vi "Post-Build Action.vi"(5 "Files Generated by Build":path[](array[path]), 6 "Top Level/Always Included VIs":path[](array[path]), 7 "Destination Path":path, 8 "error in (no error)":errorcluster, 9 "Target Name":string, 10 "Build Specification Name":string, 11 "Project Path":path) -> (0 "error out":errorcluster)   [LabVIEW 2019]
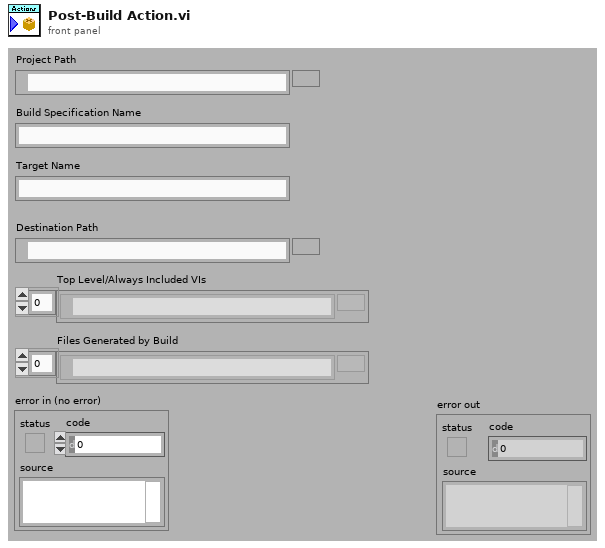
[diagram p1: front panel]
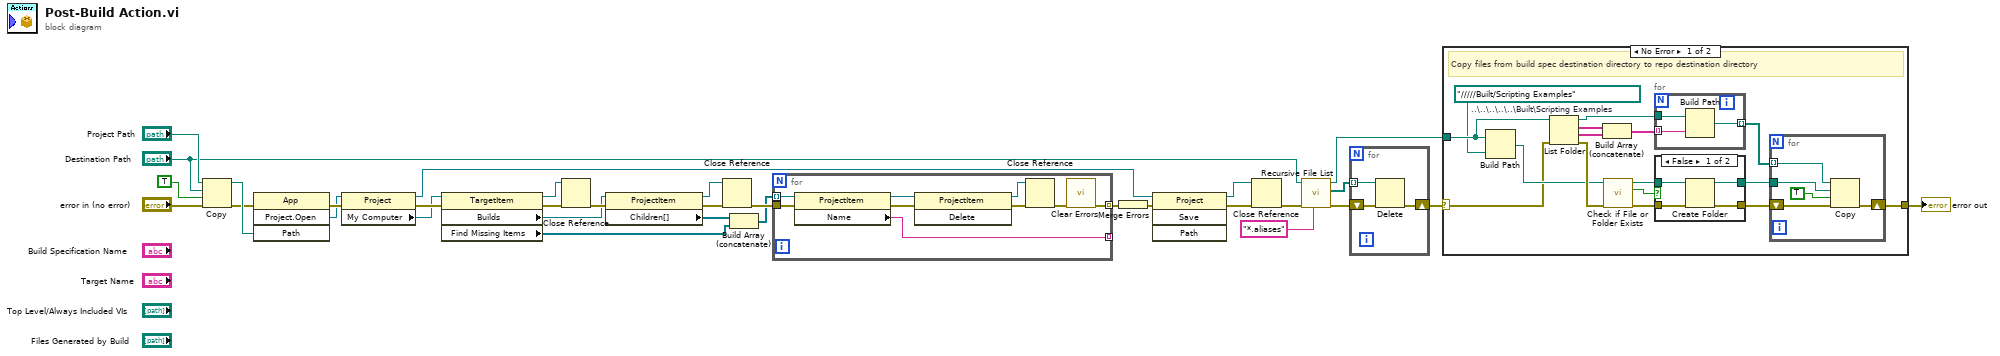
[diagram p0: block diagram]
diagram:
  n1 = Copy(8:"error in (no error)", 9:TRUE ("overwrite (F)"), 10:"Destination Path", 11:"Project Path") -> (0:w22:errorcluster, 3:w26:path)  [unwired: 1 in, 1 out]
  n2 = invoke class="App" method="Project.Open"(error in=w22, "Path"=w26) -> (error out=w23:errorcluster, "Project:Open"=w19:refnum<vi>)  [unwired: 2 in, 2 out]
  n3 = property class="Project"(reference=w19, error in=w23) -> (reference out=w25:refnum<vi>, error out=w24:errorcluster, "My Computer"=w18:refnum<vi>)
  n4 = property class="TargetItem"(reference=w18, error in=w24) -> (reference out=w6:refnum<vi>, error out=w7:errorcluster, "Builds"=w4:refnum<vi>, "Find Missing Items"=w2:refnum<vi>[])
  n5 = Close Reference(reference=w6, error in (no error)=w7) -> (error out=w5:errorcluster)
  n6 = property class="ProjectItem"(reference=w4, error in=w5) -> (reference out=w9:refnum<vi>, error out=w10:errorcluster, "Children[]"=w3:refnum<vi>[])
  n7 = Close Reference(reference=w9, error in (no error)=w10) -> (error out=w8:errorcluster)
  n8 = Build Array (concatenate)(w3, w2) -> (w1:refnum<vi>[])
  n9 = for {
    tunnel: w1 -> [w37] mode=indexing
    tunnel: [w35] -> _ mode=indexing
    tunnel: w8 -> [w39]
    tunnel: [w33] -> w11 mode=indexing
    n10 = property class="ProjectItem"(reference=w37, error in=w39) -> (reference out=w36:refnum<vi>, error out=w38:errorcluster, "Name"=w35:string)
    n11 = invoke class="ProjectItem" method="Delete"(reference=w36, error in=w38) -> (reference out=w40:refnum<vi>, error out=w41:errorcluster)  [unwired: 1 in, 1 out]
    n12 = Close Reference(reference=w40, error in (no error)=w41) -> (error out=w34:errorcluster)
    n13 = call <vilib>:"Clear Errors.vi"("error in (no error)"=w34) -> ("error out"=w33:errorcluster)  [unwired: 5 in, 1 out]
  }
  n14 = Merge Errors(w11) -> (w13:errorcluster)
  n15 = invoke class="Project" method="Save"(reference=w25, error in=w13) -> (reference out=w20:refnum<vi>, error out=w21:errorcluster)  [unwired: 2 in, 2 out]
  n16 = Close Reference(reference=w20, error in (no error)=w21) -> (error out=w17:errorcluster)
  n17 = call <vilib>:"Recursive File List.vi"("pattern"="*.aliases", "error in (no error)"=w17, "Folder Path"="Destination Path") -> ("error out"=w15:errorcluster, "All Files in Dir"=w14:path[], "dup Folder Path"=w28:path)  [unwired: 4 in, 2 out]
  n18 = for {
    shift-right: [w42] -> w27
    shift-left: w15 -> [w44]
    tunnel: w14 -> [w43] mode=indexing
    n19 = Delete(path (use dialog)=w43, error in=w44) -> (error out=w42:errorcluster)  [unwired: 3 in, 2 out]
  }
  n20 = case shown="No Error" w27 {
    selector: w27 -> [w47 w75]
    tunnel: [w58 w75] -> w12
    tunnel: w28 -> [w46 _]
    frame No Error {
      w45 = path "../../../../../Built/Scripting Examples"  # ..\..\..\..\..\Built\Scripting Examples
      # "Copy files from build spec destination directory to repo destination directory"
      n21 = Build Path(base path=w46, name or relative path=w45) -> (appended path=w53:path)
      n22 = List Folder(path=w46, error in=w47) -> (path out=w60:path, filenames=w57:string[], folder names=w56:string[], error out=w59:errorcluster)  [unwired: 2 in]
      n23 = Build Array (concatenate)(w57, w56) -> (w55:string[])
      n24 = call <vilib>:"Check if File or Folder Exists.vi"("error in (no error)"=w59, "path"=w53) -> ("error out"=w50:errorcluster, "file or folder exists?"=w52:bool, "dup path"=w51:path)  [unwired: 7 in]
      n25 = for {
        tunnel: w55 -> [w73] mode=indexing
        tunnel: w60 -> [w74]
        tunnel: [w72] -> w54 mode=indexing
        n26 = Build Path(base path=w74, name or relative path=w73) -> (appended path=w72:path)
      }
      n27 = case shown="False" w52 {
        tunnel: w51 -> [w64 w66]
        tunnel: w50 -> [w63 w65]
        tunnel: [w62 w66] -> w49
        tunnel: [w61 w65] -> w48
        frame False {
          n28 = Create Folder(path (use dialog)=w64, error in=w63) -> (created path=w62:path, error out=w61:errorcluster)  [unwired: 1 in, 1 out]
        }
        frame True {
        }
      }
      n29 = for {
        tunnel: w54 -> [w68] mode=indexing
        shift-right: [w69] -> w58
        shift-left: w48 -> [w70]
        tunnel: w49 -> [w67]
        n30 = Copy(8:w70, 9:TRUE ("overwrite (F)"), 10:w67, 11:w68) -> (0:w69:errorcluster)  [unwired: 1 in, 2 out]
      }
    }
    frame Error {
    }
  }
  "error out" <- w12
